vi "Phasor Compute Plots Product or Ratio.vi"(8 "error in (no error)":errorcluster, 9 "Operation":T1, 10 "Phasor Plot 2":cluster{"X Array":dbl[], "Y Array":dbl[]}, 11 "Phasor Plot 1":cluster{"X Array":dbl[], "Y Array":dbl[]}) -> (0 "error out":errorcluster, 1 "Metadata Phasor Plot":i32, 3 "Phasor Plot out":cluster{"X Array":dbl[], "Y Array":dbl[]})   [LabVIEW 2021, in "Phasor.lvlib"]
uses:
  Phasor Operation.ctl
  <vilib>/Utility/error.llb/Error Cluster From Error Code.vi
  <vilib>/ErrorRing/Error Ring.xnode
  Phasor.lvlib
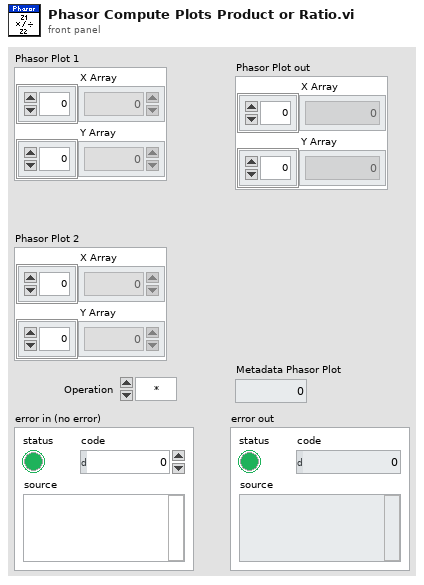
[diagram p1: front panel]
types:
  T1 = typedef "Phasor.lvlib/Phasor Operation.ctl" = enum16{"*", "/"}
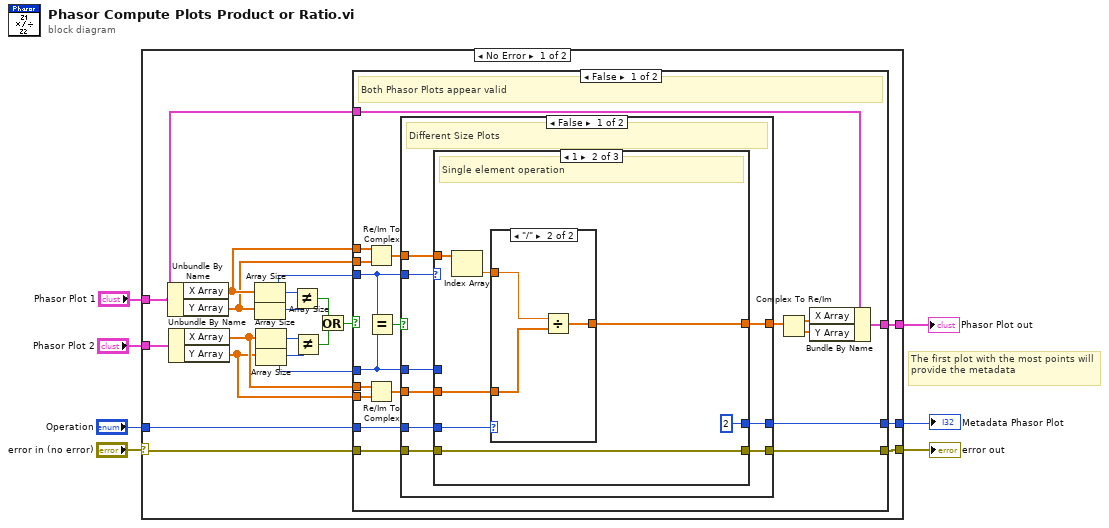
[diagram p0: block diagram]
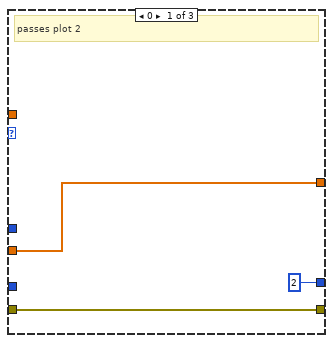
[diagram p2: hidden frame]
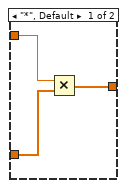
[diagram p3: hidden frame]
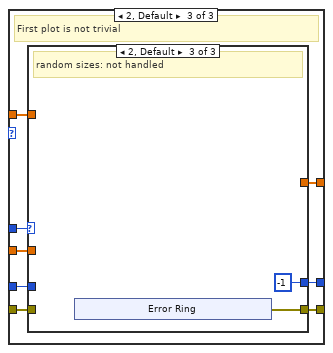
[diagram p4: hidden frame]
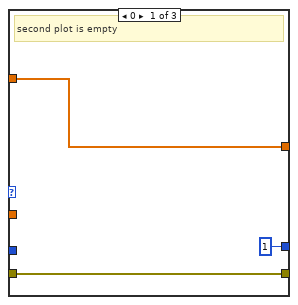
[diagram p5: hidden frame]
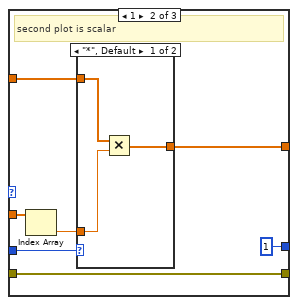
[diagram p6: hidden frame]
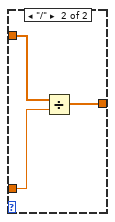
[diagram p7: hidden frame]
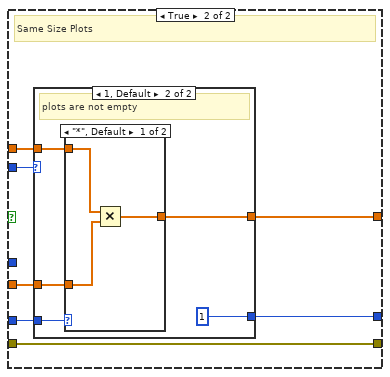
[diagram p8: hidden frame]
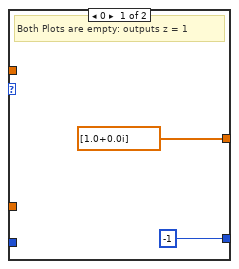
[diagram p9: hidden frame]
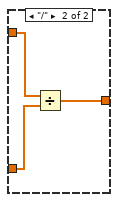
[diagram p10: hidden frame]
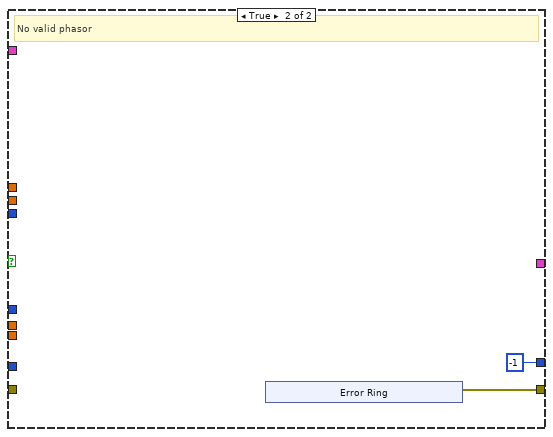
[diagram p11: hidden frame]
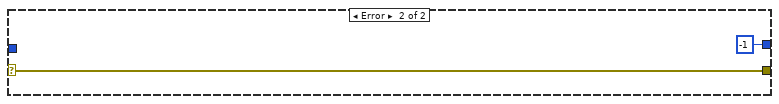
[diagram p12: hidden frame]
diagram:
  # "The first plot with the most points will provide the metadata"
  n1 = case shown="No Error" "error in (no error)" {
    selector: "error in (no error)" -> [w9 w126]
    tunnel: "Phasor Plot 1" -> [w12 _]
    tunnel: "Phasor Plot 2" -> [w23 _]
    tunnel: [w19 w126] -> w4
    tunnel: "Operation" -> [w13 _]
    tunnel: [w11 _] -> w2
    tunnel: [w8 -1 ("Ruling Phasor Plot")] -> w1
    frame No Error {
      n2 = Unbundle By Name(w12) -> ("X Array"=w16:dbl[], "Y Array"=w15:dbl[])
      n3 = Unbundle By Name(w23) -> ("X Array"=w14:dbl[], "Y Array"=w10:dbl[])
      n4 = Array Size(array=w16) -> (size(s)=w18:i32)
      n5 = Array Size(array=w15) -> (size(s)=w25:i32)
      n6 = Array Size(array=w14) -> (size(s)=w24:i32)
      n7 = Array Size(array=w10) -> (size(s)=w17:i32)
      n8 = Not Equal?(x=w18, y=w25) -> (x != y?=w22:bool)
      n9 = Not Equal?(x=w24, y=w17) -> (x != y?=w21:bool)
      n10 = Or(x=w22, y=w21) -> (x .or. y?=w20:bool)
      n11 = case shown="False" w20 {
        tunnel: [w28 w120] -> w19
        tunnel: w18 -> [w33 _]
        tunnel: w17 -> [w32 _]
        tunnel: w16 -> [w41 _]
        tunnel: w15 -> [w42 _]
        tunnel: w14 -> [w40 _]
        tunnel: w10 -> [w39 _]
        tunnel: w13 -> [w36 _]
        tunnel: w12 -> [w34 _]
        tunnel: [w35 _] -> w11
        tunnel: w9 -> [w27 _]
        tunnel: [w26 -1 ("Ruling Phasor Plot")] -> w8
        frame False {
          # "Both Phasor Plots appear valid"
          n12 = Re/Im To Complex(1:w42, 2:w41) -> (0:w37:cdb[])
          n13 = Re/Im To Complex(1:w39, 2:w40) -> (0:w38:cdb[])
          n14 = Equal?(x=w33, y=w32) -> (x = y?=w43:bool)
          n15 = case shown="False" w43 {
            tunnel: w38 -> [w51 w103]
            tunnel: w37 -> [w50 w104]
            tunnel: w36 -> [w49 w105]
            tunnel: w33 -> [w52 w102]
            tunnel: w32 -> [w47 _]
            tunnel: [w48 w101] -> w31
            tunnel: [w46 w100] -> w28
            tunnel: w27 -> [w45 w100]
            tunnel: [w44 w99] -> w26
            frame False {
              # "Different Size Plots"
              n16 = case shown="1" w52 {
                tunnel: w51 -> [w55 w59 w73]
                tunnel: w50 -> [_ w62 w74]
                tunnel: w49 -> [_ w61 w72]
                tunnel: [w55 w58 w75] -> w48
                tunnel: w47 -> [_ _ w76]
                tunnel: [w54 w57 w71] -> w46
                tunnel: w45 -> [w54 w57 w70]
                tunnel: [2 ("Ruling Phasor Plot") 2 ("Ruling Phasor Plot") w69] -> w44
                frame 0 {
                  # "passes plot 2"
                }
                frame 1 {
                  # "Single element operation"
                  n17 = Index Array(array=w62) -> (element=w60:cdb)  [unwired: 1 in]
                  n18 = case shown="\"/\"" w61 {
                    tunnel: w60 -> [w65 w68]
                    tunnel: w59 -> [w64 w67]
                    tunnel: [w63 w66] -> w58
                    frame "*", Default {
                      n19 = Multiply(x=w65, y=w64) -> (x*y=w63:cdb[])
                    }
                    frame "/" {
                      n20 = Divide(x=w68, y=w67) -> (x/y=w66:cdb[])
                    }
                  }
                }
                frame 2, Default {
                  # "First plot is not trivial"
                  n21 = case shown="2, Default" w76 {
                    tunnel: [w79 w82 _] -> w75
                    tunnel: w74 -> [w79 w84 _]
                    tunnel: w73 -> [_ w86 _]
                    tunnel: w72 -> [_ w85 _]
                    tunnel: [w78 w81 w94] -> w71
                    tunnel: w70 -> [w78 w81 _]
                    tunnel: [1 ("Ruling Phasor Plot") 1 ("Ruling Phasor Plot") -1 ("Ruling Phasor Plot")] -> w69
                    frame 0 {
                      # "second plot is empty"
                    }
                    frame 1 {
                      # "second plot is scalar"
                      n22 = Index Array(array=w86) -> (element=w83:cdb)  [unwired: 1 in]
                      n23 = case shown="\"*\", Default" w85 {
                        tunnel: w84 -> [w89 w92]
                        tunnel: w83 -> [w88 w91]
                        tunnel: [w87 w90] -> w82
                        frame "*", Default {
                          n24 = Multiply(x=w89, y=w88) -> (x*y=w87:cdb[])
                        }
                        frame "/" {
                          n25 = Divide(x=w92, y=w91) -> (x/y=w90:cdb[])
                        }
                      }
                    }
                    frame 2, Default {
                      # "random sizes: not handled"
                      n26 = xnode "Error Ring"() -> ("error out"=w94:errorcluster)
                    }
                  }
                }
              }
            }
            frame True {
              # "Same Size Plots"
              n27 = case shown="1, Default" w102 {
                tunnel: w105 -> [_ w112]
                tunnel: w104 -> [_ w111]
                tunnel: w103 -> [_ w110]
                tunnel: [cdb[] [1.0+0.0i] w109] -> w101
                tunnel: [-1 ("Ruling Phasor Plot") 1 ("Ruling Phasor Plot")] -> w99
                frame 0 {
                  # "Both Plots are empty: outputs z = 1"
                }
                frame 1, Default {
                  # "plots are not empty"
                  n28 = case shown="\"*\", Default" w112 {
                    tunnel: w111 -> [w115 w118]
                    tunnel: w110 -> [w114 w117]
                    tunnel: [w113 w116] -> w109
                    frame "*", Default {
                      n29 = Multiply(x=w115, y=w114) -> (x*y=w113:cdb[])
                    }
                    frame "/" {
                      n30 = Divide(x=w118, y=w117) -> (x/y=w116:cdb[])
                    }
                  }
                }
              }
            }
          }
          n31 = Complex To Re/Im(x + iy=w31) -> (x=w30:dbl[], y=w29:dbl[])
          n32 = Bundle By Name(cluster=w34, "X Array"=w30, "Y Array"=w29) -> (w35:cluster{"X Array":dbl[], "Y Array":dbl[]})
        }
        frame True {
          # "No valid phasor"
          n33 = xnode "Error Ring"() -> ("error out"=w120:errorcluster)
        }
      }
    }
    frame Error {
    }
  }
  "error out" <- w4
  "Phasor Plot out" <- w2
  "Metadata Phasor Plot" <- w1
